vi "Gimbal control.vi"(0 "Position 5":dbl, 1 "output cluster":T26 {"A/SPI - LiDAR"."SPI Configuration"."Frame Length" min=1 max=16}, 2 "Particle Measurements (Pixels)":dbl[][](array[numeric]), 3 "element":bool, 5 "error in (no error)":errorcluster, 6 "Position 3":dbl) -> (12 "Position 2":dbl, 13 "Antal isbjerg":i32, 14 "PWM Ref Out 2":T1, 15 "PWM Ref Out":T1, 16 "Position 4":dbl, 17 "Y":dbl[](array[numeric]), 18 "X":dbl[](array[numeric]), 19 "error out":errorcluster)   [LabVIEW 2018]
uses:
  <vilib>/myRIO/Instrument Drivers/Onboard IO/DIO/typedefs/DIO Reference.ctl
  <vilib>/myRIO/Common/Instrument Driver Framework/Utilities/typedefs/myRIO Generic Hardware Reference.ctl
  <vilib>/myRIO/Common/Instrument Driver Framework/Utilities/typedefs/Hardware Version Enum.ctl
  <vilib>/myRIO/Common/Instrument Driver Framework/Utilities/typedefs/myRIO v1.0 Reference.ctl
  <vilib>/myRIO/Common/Instrument Driver Framework/Utilities/typedefs/Generic FPGA Reference.ctl
  <vilib>/myRIO/Common/Instrument Driver Framework/myRIO v1.0/DIO/typedefs/DIO Channels List.ctl
  <vilib>/myRIO/Common/Instrument Driver Framework/myRIO v1.0/DIO/typedefs/DIO Channels Enum.ctl
  <vilib>/myRIO/Instrument Drivers/Onboard IO/PWM/typedefs/PWM Reference.ctl
  <vilib>/myRIO/Common/Instrument Driver Framework/myRIO v1.0/PWM/typedefs/PWM Channels Enum.ctl
  <vilib>/myRIO/Instrument Drivers/Onboard IO/PWM/typedefs/PWM Configuration.ctl
  <vilib>/myRIO/Instrument Drivers/Onboard Devices/Accelerometer/typedefs/Accelerometer Reference.ctl
  <vilib>/myRIO/Common/Instrument Driver Framework/myRIO v1.0/Accelerometer/typedefs/Accelerometer Channels List.ctl
  <vilib>/myRIO/Common/Instrument Driver Framework/myRIO v1.0/Accelerometer/typedefs/Accelerometer Channels Enum.ctl
  <vilib>/myRIO/Instrument Drivers/Onboard IO/AI/typedefs/AI Reference.ctl
  <vilib>/myRIO/Common/Instrument Driver Framework/myRIO v1.0/AI/typedefs/AI Channels List.ctl
  <vilib>/myRIO/Common/Instrument Driver Framework/myRIO v1.0/AI/typedefs/AI Channels Enum.ctl
  <vilib>/myRIO/Common/Instrument Driver Framework/Utilities/typedefs/Analog Scaling Constants List.ctl
  <vilib>/myRIO/Common/Instrument Driver Framework/Utilities/typedefs/Analog Scaling Constants.ctl
  <vilib>/myRIO/Instrument Drivers/Onboard IO/SPI/typedefs/SPI Reference.ctl
  <vilib>/myRIO/Common/Instrument Driver Framework/myRIO v1.0/SPI/typedefs/SPI Channels Enum.ctl
  <vilib>/myRIO/Instrument Drivers/Onboard IO/SPI/typedefs/SPI Configuration.ctl
  <vilib>/myRIO/Common/Instrument Driver Framework/myRIO v1.0/SPI/typedefs/SPI Clock Phase.ctl
  <vilib>/myRIO/Common/Instrument Driver Framework/myRIO v1.0/SPI/typedefs/SPI Clock Polarity.ctl
  <vilib>/myRIO/Common/Instrument Driver Framework/myRIO v1.0/SPI/typedefs/SPI Data Direction.ctl
  <vilib>/myRIO/Common/Instrument Driver Framework/myRIO v1.0/SPI/typedefs/SPI Frame Length.ctl
  <vilib>/Utility/error.llb/Error Cluster From Error Code.vi
  <vilib>/myRIO/Common/Instrument Driver Framework/myRIO v1.0/PWM/vis/myRIO v1.0 Write PWM.vi
  <vilib>/myRIO/Instrument Drivers/Onboard IO/PWM/PWM.lvlib
  <vilib>/myRIO/Instrument Drivers/Onboard IO/DIO/DIO.lvlib
  <vilib>/myRIO/Instrument Drivers/Onboard Devices/Accelerometer/Accelerometer.lvlib
  <vilib>/myRIO/Instrument Drivers/Onboard IO/AI/AI.lvlib
  <vilib>/myRIO/Instrument Drivers/Onboard IO/SPI/SPI.lvlib
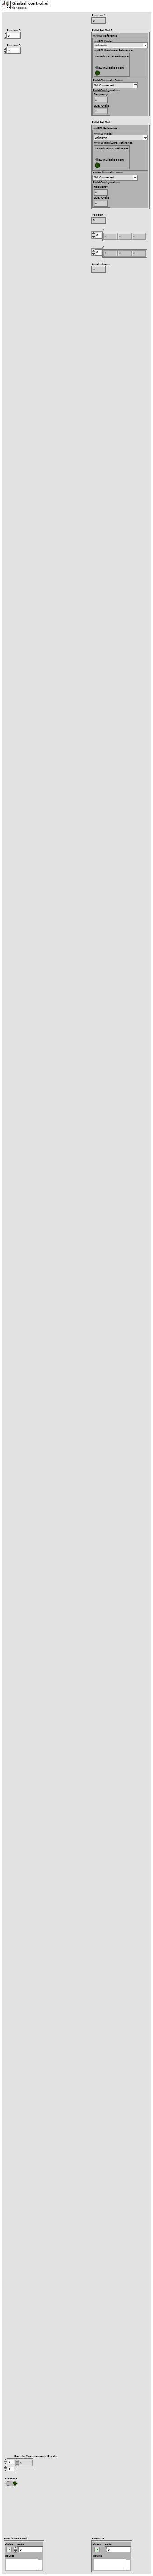
[diagram p1: front panel]
types:
  T1 = typedef "PWM.lvlib/PWM Reference.ctl" = cluster{"myRIO Reference":T2, "PWM Channels Enum":T6, "PWM Configuration":T7}
  T2 = typedef "myRIO Generic Hardware Reference.ctl" = cluster{"myRIO Model":T3, "myRIO Hardware Reference":T4}
  T3 = typedef "Hardware Version Enum.ctl" = enum16{"Unknown", "myRIO-1900", "myRIO-1950", "roboRIO", "NI ELVIS RIO CM", "ELVIS III"}
  T4 = typedef "myRIO v1.0 Reference.ctl" = cluster{"Generic FPGA Reference":T5, "Allow multiple opens":bool}
  T5 = typedef "Generic FPGA Reference.ctl" = refnum<k20>
  T6 = typedef "PWM Channels Enum.ctl" = enum16{"Not Connected", "C/PWM0", "C/PWM1", "A/PWM0", "A/PWM1", "A/PWM2", "A/PWM3", "A/PWM4", "A/PWM5", "A/PWM6", "A/PWM7", "A/PWM8", "A/PWM9", "A/PWM10", "A/PWM11", "A/PWM12", "A/PWM13", "A/PWM14", "A/PWM15", "A/PWM16", "A/PWM17", "A/PWM18", "A/PWM19", "B/PWM0", "B/PWM1", "B/PWM2", "B/PWM3", "B/PWM4", "B/PWM5", "B/PWM6", "B/PWM7", "B/PWM8", "B/PWM9", "B/PWM10", "B/PWM11", "B/PWM12", "B/PWM13", "B/PWM14", "B/PWM15", "B/PWM16", "B/PWM17", "B/PWM18", "B/PWM19", "PWM/PWM0", "PWM/PWM1", "PWM/PWM2", "PWM/PWM3", "PWM/PWM4", "PWM/PWM5", "PWM/PWM6", "PWM/PWM7", "PWM/PWM8", "PWM/PWM9"}
  T7 = typedef "PWM.lvlib/PWM Configuration.ctl" = cluster{"Frequency":dbl, "Duty Cycle":dbl}
  T8 = typedef "DIO.lvlib/DIO Reference.ctl" = cluster{"myRIO Reference":T2, "DIO Channels List":T9}
  T9 = typedef "DIO Channels List.ctl" = T10[]
  T10 = typedef "DIO Channels Enum.ctl" = enum16{"Not Connected", "C/DIO0", "C/DIO1", "C/DIO2", "C/DIO3", "C/DIO4", "C/DIO5", "C/DIO6", "C/DIO7", "A/DIO0", "A/DIO1", "A/DIO2", "A/DIO3", "A/DIO4", "A/DIO5", "A/DIO6", "A/DIO7", "A/DIO8", "A/DIO9", "A/DIO10", "A/DIO11", "A/DIO12", "A/DIO13", "A/DIO14", "A/DIO15", "A/DIO16", "A/DIO17", "A/DIO18", "A/DIO19", "B/DIO0", "B/DIO1", "B/DIO2", "B/DIO3", "B/DIO4", "B/DIO5", "B/DIO6", "B/DIO7", "B/DIO8", "B/DIO9", "B/DIO10", "B/DIO11", "B/DIO12", "B/DIO13", "B/DIO14", "B/DIO15", "B/DIO16", "B/DIO17", "B/DIO18", "B/DIO19", "LED0", "LED1", "LED2", "LED3", "Button0", "DIO/DIO0", "DIO/DIO1", "DIO/DIO2", "DIO/DIO3", "DIO/DIO4", "DIO/DIO5", "DIO/DIO6", "DIO/DIO7", "DIO/DIO8", "DIO/DIO9", "SPI/CS0", "SPI/CS1", "SPI/CS2", "SPI/CS3", "LED RADIO (Green)", "LED RADIO (Red)", "LED COMM (Green)", "LED COMM (Red)", "LED MODE (Green)", "LED MODE (Red)"}
  T11 = typedef "Accelerometer.lvlib/Accelerometer Reference.ctl" = cluster{"myRIO Reference":T2, "Accelerometer Channels List":T12, "LSB Weight":dbl}
  T12 = typedef "Accelerometer Channels List.ctl" = T13[]
  T13 = typedef "Accelerometer Channels Enum.ctl" = enum16{"Not Connected", "X-Axis", "Y-Axis", "Z-Axis"}
  T14 = typedef "AI.lvlib/AI Reference.ctl" = cluster{"myRIO Reference":T2, "AI Channels List":T15, "AI Scaling Constants List":T17}
  T15 = typedef "AI Channels List.ctl" = T16[]
  T16 = typedef "AI Channels Enum.ctl" = enum16{"Not Connected", "AudioIn/Left", "AudioIn/Right", "C/AI0", "C/AI1", "A/AI0", "A/AI1", "A/AI2", "A/AI3", "A/AI4", "A/AI5", "A/AI6", "A/AI7", "B/AI0", "B/AI1", "B/AI2", "B/AI3", "B/AI4", "B/AI5", "B/AI6", "B/AI7", "AI/AI0", "AI/AI1", "AI/AI2", "AI/AI3", "A/AI0 (DIFF)", "A/AI1 (DIFF)", "A/AI2 (DIFF)", "A/AI3 (DIFF)", "B/AI0 (DIFF)", "B/AI1 (DIFF)", "B/AI2 (DIFF)", "B/AI3 (DIFF)"}
  T17 = typedef "Analog Scaling Constants List.ctl" = T18[]
  T18 = typedef "Analog Scaling Constants.ctl" = cluster{"LSB Weight (Volts)":dbl, "Offset (Volts)":dbl, "Signed?":bool}
  T19 = typedef "SPI.lvlib/SPI Reference.ctl" = cluster{"myRIO Reference":T2, "SPI Channels Enum":T20, "SPI Configuration":T21}
  T20 = typedef "SPI Channels Enum.ctl" = enum16{"Not Connected", "A/SPI", "B/SPI", "SPI/SPI"}
  T21 = typedef "SPI.lvlib/SPI Configuration.ctl" = cluster{"Frequency [Hz]":dbl, "Clock Phase":T22, "Clock Polarity":T23, "Data Direction":T24, "Frame Length":T25}
  T22 = typedef "SPI Clock Phase.ctl" = enum8{"Leading", "Trailing"}
  T23 = typedef "SPI Clock Polarity.ctl" = enum8{"Low", "High"}
  T24 = typedef "SPI Data Direction.ctl" = enum8{"Most significant bit first", "Least significant bit first"}
  T25 = typedef "SPI Frame Length.ctl" = u8
  T26 = cluster{"B/DIO0 - Stepper Direction":T8, "B/DIO1 - Stepper1 Enable":T8, "B/DIO2 - Stepper2 Enable":T8, "B/DIO3 - Stepper3 Enable":T8, "B/DIO4 - Endstop Stepper1 Top":T8, "B/DIO11 - Endstop Stepper1 Bund":T8, "B/DIO12 - Endstop Stepper2 Top":T8, "B/DIO13 - Endstop Stepper2 Bund":T8, "B/DIO14 - Endstop Stepper3 Top":T8, "B/DIO15 - Endstop Stepper3 Bund":T8, "A/DIO0 - Cooler":T8, "A/DIO1 - Beacon drop (dio1)":T8, "A/DIO2 - Beacon drop (dio0)":T8, "A/DIO3 - QuickRelease (dio1)":T8, "A/DIO4 - QuickRelease (dio0)":T8, "A/DIO11 - LiDAR SPI CS":T8, "B/PWM0 - Stepper":T1, "B/PWM1 - Drill":T1, "A/PWM0 - Servo_Roll":T1, "A/PWM1 - Servo_Yaw":T1, "Acc. X-axis":T11, "Acc. Y-axis":T11, "B/AI0 - Drone Grounded F3":T14, "B/AI1 - Drone Drill Gear F4":T14, "B/AI2 - Beacon Drop F5":T14, "B/AI3 - Drone Drill Boost F6":T14, "A/AI0 - Drone Stepper F8":T14, "A/AI1 - Beacon Wiper":T14, "A/AI2 - QuickRelease Wiper":T14, "A/AI3 - Drill Current":T14, "A/SPI - LiDAR":T19, "B/UART - XBee":refnum<visa-resource-name>, "A/UART - A3 GPS":refnum<visa-resource-name>, "RIO Flashing LEDs":T8}
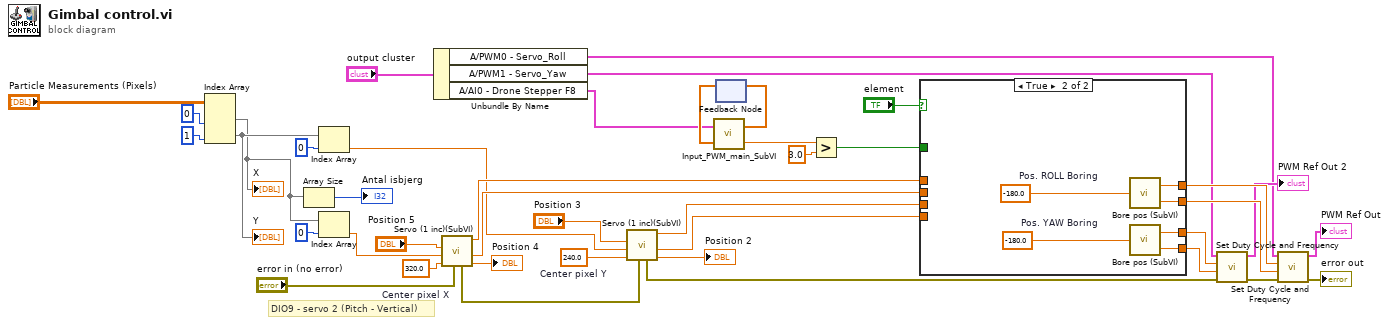
[diagram p0: block diagram]
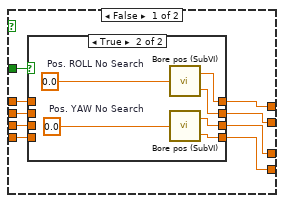
[diagram p2: hidden frame]
diagram:
  w13 = 240.0  # Center pixel Y
  w3 = 320.0  # Center pixel X
  # "DIO9 - servo 2 (Pitch - Vertical)"
  n1 = Index Array(array="Particle Measurements (Pixels)", index (col) #1=0 ("index (col)"), index (col) #2=1 ("index (col)")) -> (element #1=w8:dbl[], element #2=w11:dbl[])  [unwired: 2 in]
  "Y" <- w11
  "X" <- w8
  n2 = Array Size(array=w8) -> (size(s)=→"Antal isbjerg":i32)
  n3 = Index Array(array=w11, index=0) -> (element=w16:dbl)
  n4 = Index Array(array=w8, index=0) -> (element=w9:dbl)
  n5 = Unbundle By Name("output cluster") -> ("A/PWM0 - Servo_Roll"=w20:T1, "A/PWM1 - Servo_Yaw"=w19:T1, "A/AI0 - Drone Stepper F8"=w36:T14)
  n6 = call "Servo (1 inc)(SubVI).vi"("error constant 2"="error in (no error)", "Center pixel"=w3, "Pixel value"=w9, "Position."="Position 5") -> ("Position 2"=→"Position 4":dbl, "freq [Hz]"=w35:dbl, "Duty"=w31:dbl, "error constant"=w14:errorcluster)  [unwired: 3 in, 1 out]
  n7 = call "Servo (1 inc)(SubVI).vi"("error constant 2"=w14, "Center pixel"=w13, "Pixel value"=w16, "Position."="Position 3") -> ("Position 2"=→"Position 2":dbl, "freq [Hz]"=w33:dbl, "Duty"=w29:dbl, "error constant"=w24:errorcluster)  [unwired: 3 in, 1 out]
  n8 = feedback #1() -> (w38:dbl[])  [unwired: 1 in]
  n9 = call "Input_PWM_main_SubVI.vi"("Shift in"=w38, "AI Ref In"=w36) -> ("Value out"=w39:dbl, "Shift out"=w37:dbl[])
  n10 = feedback-in #1(w37) -> ()
  n11 = Greater?(x=w39, y=3.0) -> (0:w41:bool)
  n12 = case shown="True" "element" {
    tunnel: [w48 w65] -> w28
    tunnel: w29 -> [w47 _]
    tunnel: [w46 w66] -> w30
    tunnel: w31 -> [w45 _]
    tunnel: [w50 w64] -> w32
    tunnel: w33 -> [w49 _]
    tunnel: [w44 w63] -> w34
    tunnel: w35 -> [w43 _]
    tunnel: w41 -> [w42 _]
    frame False {
      n13 = case shown="True" w42 {
        tunnel: [w54 w57] -> w50
        tunnel: w49 -> [w54 _]
        tunnel: [w53 w56] -> w48
        tunnel: w47 -> [w53 _]
        tunnel: [w52 w55] -> w46
        tunnel: w45 -> [w52 _]
        tunnel: [w51 w58] -> w44
        tunnel: w43 -> [w51 _]
        frame False {
        }
        frame True {
          w60 = 0.0  # Pos. YAW No Search
          w59 = 0.0  # Pos. ROLL No Search
          n14 = call "Bore pos (SubVI).vi"("Position."=w59) -> ("Duty"=w55:dbl, "freq [Hz]"=w58:dbl)
          n15 = call "Bore pos (SubVI).vi"("Position."=w60) -> ("Duty"=w56:dbl, "freq [Hz]"=w57:dbl)
        }
      }
    }
    frame True {
      w62 = -180.0  # Pos. YAW Boring
      w61 = -180.0  # Pos. ROLL Boring
      n16 = call "Bore pos (SubVI).vi"("Position."=w61) -> ("Duty"=w66:dbl, "freq [Hz]"=w63:dbl)
      n17 = call "Bore pos (SubVI).vi"("Position."=w62) -> ("Duty"=w65:dbl, "freq [Hz]"=w64:dbl)
    }
  }
  n18 = call <vilib>:"Set Duty Cycle and Frequency.vi"("error in (no error)"=w24, "Frequency [Hz]"=w32, "Duty Cycle"=w28, "PWM Ref In"=w19) -> ("error out"=w25:errorcluster, "PWM Ref Out"=→"PWM Ref Out 2":T1)  [unwired: 5 in]
  n19 = call <vilib>:"Set Duty Cycle and Frequency.vi"("error in (no error)"=w25, "Frequency [Hz]"=w34, "Duty Cycle"=w30, "PWM Ref In"=w20) -> ("error out"=→"error out":errorcluster, "PWM Ref Out"=→"PWM Ref Out":T1)  [unwired: 5 in]
